vi "WINDOW_TITLE.vi"(0 "VISA IN":refnum<visa-resource-name>, 1 "ON | OFF":bool, 2 "Title":string, 5 "error in":errorcluster, 7 "Window":i32=1) -> (14 "VISA Out":refnum<visa-resource-name>, 19 "error out":errorcluster)   [LabVIEW 2018, in "PNA-X.lvlib"]
uses:
  PNA-X.lvlib
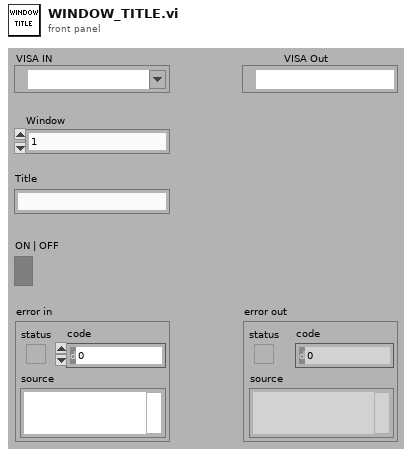
[diagram p1: front panel]
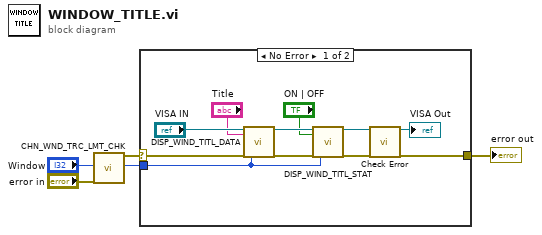
[diagram p0: block diagram]
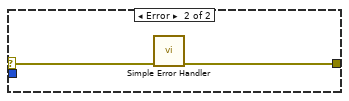
[diagram p2: hidden frame]
diagram:
  n1 = call "CHN_WND_TRC_LMT_CHK.vi"("Window"="Window", "error in"="error in") -> ("error out"=w2:errorcluster, "Window"=w1:i32)  [unwired: 13 in, 3 out]
  n2 = case shown="No Error" w2 {
    selector: w2 -> [w14 w18]
    tunnel: [w16 w17] -> w4
    tunnel: w1 -> [w8 _]
    frame No Error {
      n3 = call "DISP_WIND_TITL_DATA.vi"("VISA IN"="VISA IN", "Title"="Title", "error in"=w14, "Window"=w8) -> ("VISA Out"=w10:refnum<visa-resource-name>, "error out"=w13:errorcluster)  [unwired: 14 in]
      n4 = call "DISP_WIND_TITL_STAT.vi"("VISA IN"=w10, "ON | OFF"="ON | OFF", "error in"=w13, "Window"=w8) -> ("VISA Out"=w9:refnum<visa-resource-name>, "error out"=w12:errorcluster)  [unwired: 14 in]
      n5 = call "Check Error.vi"("VISA Resource Name"=w9, "error in (no error)"=w12) -> ("dup VISA session"=→"VISA Out":refnum<visa-resource-name>, "error out"=w16:errorcluster)  [unwired: 16 in]
    }
    frame Error {
      n6 = call <vilib>:"Simple Error Handler.vi"("error in (no error)"=w18) -> ("error out"=w17:errorcluster)  [unwired: 4 in, 4 out]
    }
  }
  "error out" <- w4
